vi "Default Settings.vi"(8 "error in (no error)":errorcluster, 10 "Module In":refnum<class "Module.lvclass">, 11 "Syringe Space in":refnum<class "Syringe Space.lvclass">) -> (0 "error out":errorcluster, 2 "Module Out":refnum<class "Module.lvclass">, 3 "Syringe Space out":refnum<class "Syringe Space.lvclass">)   [LabVIEW 2021, in "Syringe Space.lvclass"]
uses:
  Syringe Space.lvclass
  C:/Users/HEP/Documents/GitHub/UCSB-Gantry-HEP/Classes/Workspace/Carrier Tray/Assembly Tray.lvclass
  Module/Module.lvclass
  Assembly Tray.lvclass/Assembly Tray.ctl
  Write Syringe.vi
  Assembly Tray.lvclass
  Syringe Space.lvclass/Syringe Space.ctl
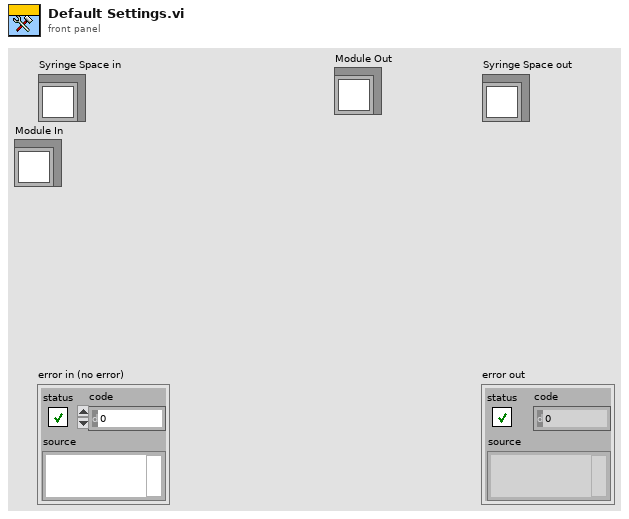
[diagram p1: front panel]
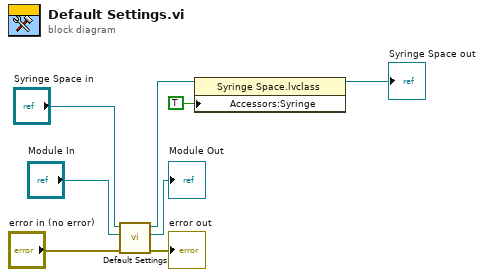
[diagram p0: block diagram]
diagram:
  n1 = call-parent "Default Settings.vi"("error in (no error)"="error in (no error)", "Module In"="Module In", "Carrier Tray in"="Syringe Space in") -> ("error out"=→"error out":errorcluster, "Module Out"=→"Module Out":refnum<class "Module.lvclass">, "Carrier Tray out"=w2:refnum<class "Syringe Space.lvclass">)  [unwired: 6 in]
  n2 = property class="Syringe Space.lvclass"(reference=w2, "Accessors:Syringe"=TRUE ("Syringe")) -> (reference out=→"Syringe Space out":refnum<class "Syringe Space.lvclass">)  [unwired: 1 in, 1 out]
